vi "runTestScenario.vi"(8 "error in (no error)":errorcluster, 11 "ADC Channel0 Test  in":refnum<class "ADC Channel0 Test.lvclass">) -> (0 "error out":errorcluster, 1 "Result":T1, 2 "TestExecution":T2, 3 "ADC Channel0 Test  out":refnum<class "ADC Channel0 Test.lvclass">)   [LabVIEW 2015, in "ADC Channel0 Test.lvclass"]
uses:
  ADC Channel0 Test.lvclass
  Typedefs/TestExecution.ctl
  Typedefs/PassFailTest.ctl
  ADC Channel0 Test.lvclass/ADC Channel0 Test.ctl
  Typedefs/WriteDataFileInput.ctl
  Typedefs/TestScenarioTypes.ctl
  Typedefs/WriteLogMessageInput.ctl
  <userlib>/Common/ILC/ILC/ILC.lvclass/ILC.ctl
  Model/TestLog/ITestLog/ITestLog.lvclass
  Typedefs/ILCBTTypedefs.lvlib
  <userlib>/Common/ILC/ILC/ILC.lvclass
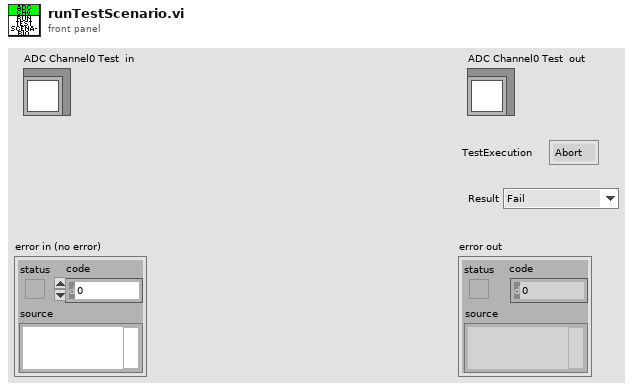
[diagram p1: front panel]
types:
  T1 = typedef "ILCBTTypedefs.lvlib/PassFailTest.ctl" = enum16{"Fail", "Pass", "NA"}
  T2 = typedef "ILCBTTypedefs.lvlib/TestExecution.ctl" = enum16{"Abort", "Continue"}
  T3 = typedef "ILCBTTypedefs.lvlib/WriteLogMessageInput.ctl" = cluster{"Test Scenario":T4, "Description":string, "Actual Value":string, "Data File":string, "Result":T1}
  T4 = typedef "ILCBTTypedefs.lvlib/TestScenarioTypes.ctl" = enum16{"+3.3VA Supply Test", "+3.3VD Supply Test", "+5VA Supply Test", "+5VD Supply Test", "Unique ID Test", "TEDS Status Test", "LIMSW1_TTL Low Test", "LIMSW1_TTL High Test", "LIMSW2_TTL Low Test", "LIMSW2_TTL High Test", "Tachometer Low Test", "Tachometer High Test", "SSR_TTL Low Test", "SSR_TTL High Test", "SM_GPI Low Test", "SM_GPI High Test", "CW Motion Without Limit Test", "CW Motion With Limit Test", "CW Motion With Both Limits Test", "CW Motion on CCW Limit Test", "CCW Motion Without Limit Test", "CCW Motion With Limit Test", "CCW Motion With Both Limits Test", "CCW Motion on CW Limit Test", "RS232-TXD Low Test", "RS232-TXD High Test", "RS232-RTS Low Test", "RS232-RTS High Test", "RS232-RXD Low Test", "RS232-RXD High Test", "RS232-CTS Low Test", "RS232-CTS High Test", "Out_SS Low Test", "Out_SS High Test", "Out_SDI Low Test", "Out_SDI High Test", "Out_SCLK Low Test", "Out_SCLK High Test", "Reset Low Test", "Reset High Test", "1 Channel ADC Test", "3 Channel ADC Test", "5 Channel ADC Test", "Vref Test", "ROT Test", "DAC1 Test", "DAC2 Test", "DAC3 Test", "DAC4 Test", "BIAS Test", "EXC1 Test", "EXC2 Test", "EXC3 Test", "EXC4 Test"}
  T5 = typedef "ILCBTTypedefs.lvlib/WriteDataFileInput.ctl" = cluster{"Test Scenario":T4, "File Name":string, "Output":string[]}
  T6 = typedef "ILCCommon.lvlib/ILCTypedefs.lvlib/InputData.ctl" = cluster{"Input Channels":T7, "Limit Switches":T8, "Tachometer":u16, "SSI Encoder":i32, "ADCs":T9}
  T7 = typedef "ILCCommon.lvlib/ILCConfiguration.lvlib/InputChannels.ctl" = enum16{"Channel 0", "3 Channels", "5 Channels"}
  T8 = typedef "ILCCommon.lvlib/ILCTypedefs.lvlib/LimitSwitches.ctl" = cluster{"1":bool, "2":bool}
  T9 = typedef "ILCCommon.lvlib/ILCTypedefs.lvlib/ADCs.ctl" = cluster{"Ch0":i32, "Ch1":i32, "Ch2":i32, "Ch3":i32, "Ch4":i32}
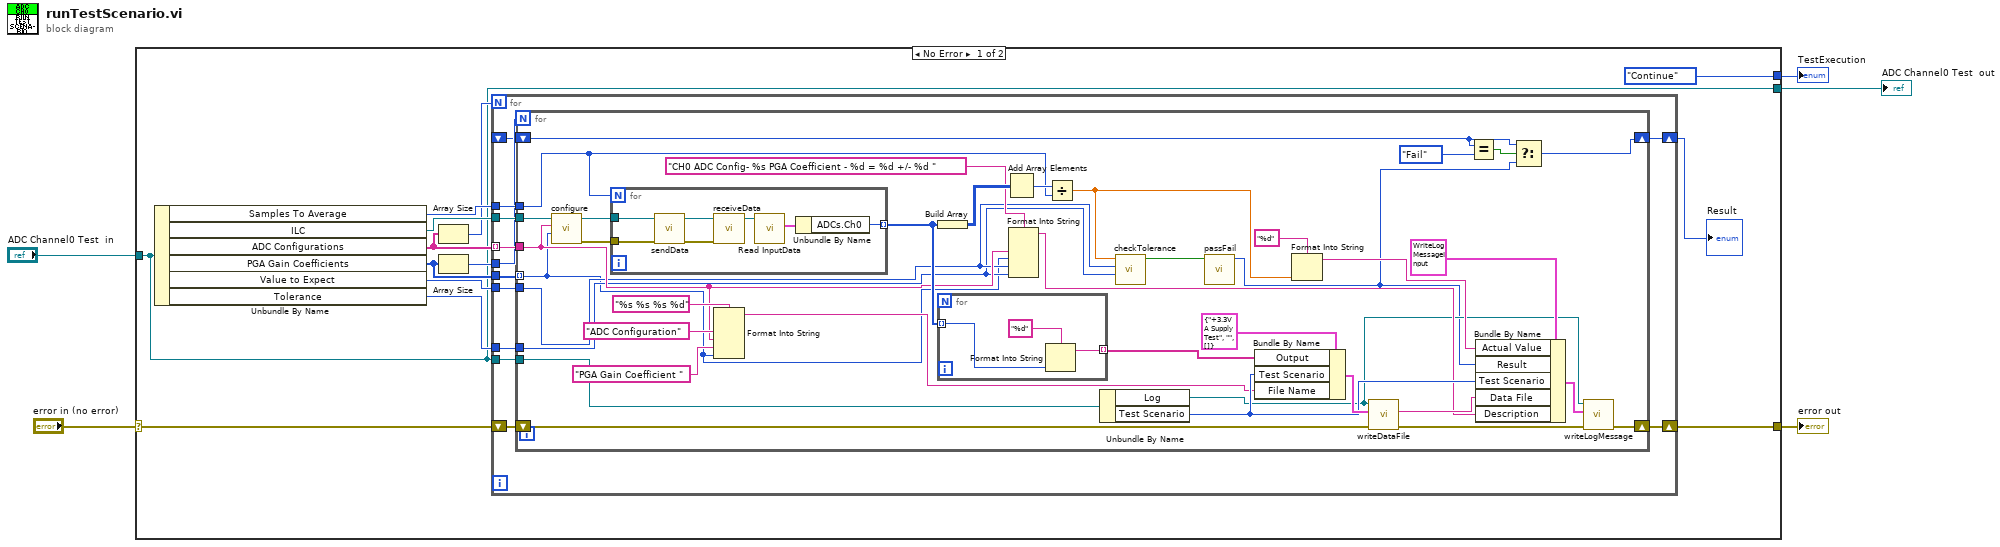
[diagram p0: block diagram]
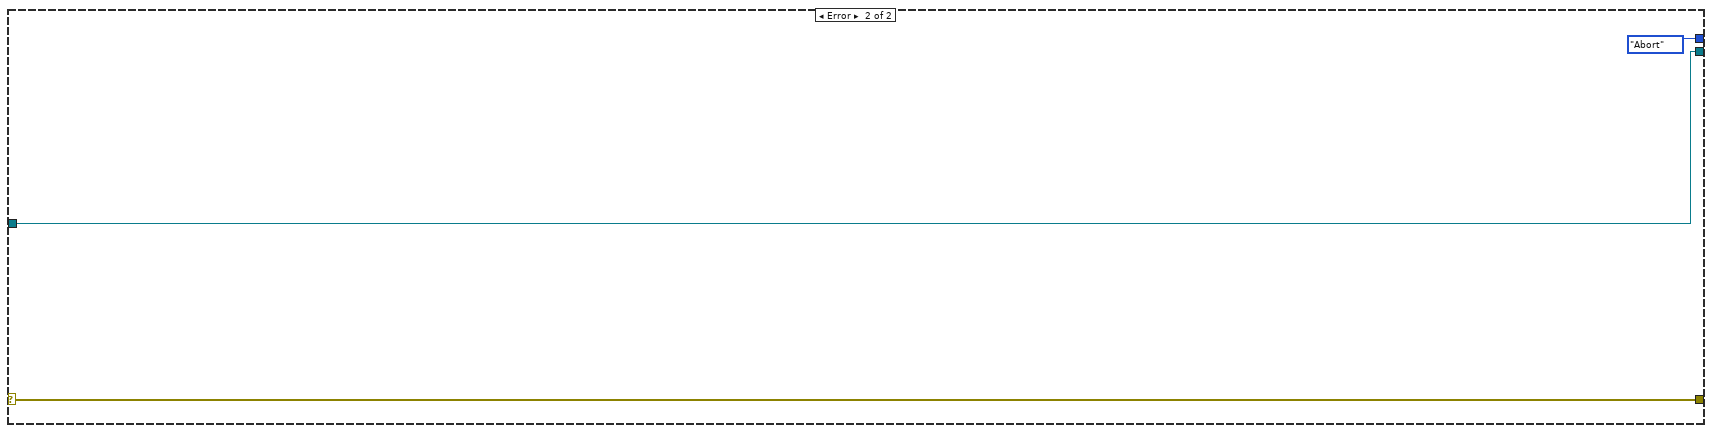
[diagram p2: hidden frame]
diagram:
  n1 = case shown="No Error" "error in (no error)" {
    selector: "error in (no error)" -> [w13 w81]
    tunnel: [w12 w81] -> w4
    tunnel: [TestExecution."Continue" ("TestExecution") TestExecution."Abort" ("TestExecution")] -> w3
    tunnel: "ADC Channel0 Test  in" -> [w7 w79]
    tunnel: [w7 w79] -> w1
    frame No Error {
      n2 = Unbundle By Name(w7) -> ("Samples To Average"=w16:i32, "ILC"=w18:refnum<class "ILC.lvclass">, "ADC Configurations"=w11:string[], "PGA Gain Coefficients"=w9:u16[], "Value to Expect"=w15:i32, "Tolerance"=w14:i32)
      n3 = Array Size(array=w11) -> (size(s)=w10:i32)
      n4 = Array Size(array=w9) -> (size(s)=w8:i32)
      n5 = for {
        N: w10 -> [_]
        tunnel: w18 -> [w30]
        tunnel: w9 -> [w21]
        tunnel: w16 -> [w29]
        tunnel: w7 -> [w28]
        tunnel: w15 -> [w27]
        tunnel: w14 -> [w26]
        tunnel: w11 -> [w23] mode=indexing
        shift-right: [w24] -> w12
        shift-left: w13 -> [w25]
        tunnel: w8 -> [w22]
        shift-right: [w20] -> w6
        shift-left: _ -> [w19]
        n6 = for {
          N: w22 -> [_]
          tunnel: w30 -> [w68]
          tunnel: w29 -> [w64]
          tunnel: w28 -> [w56]
          tunnel: w27 -> [w47]
          tunnel: w26 -> [w46]
          shift-right: [w37] -> w24
          shift-left: w25 -> [w39]
          tunnel: w23 -> [w48]
          tunnel: w21 -> [w36] mode=indexing
          shift-right: [w33] -> w20
          shift-left: w19 -> [w32]
          n7 = call <userlib>:"configure.vi"("PGA Gain"=w36, "ADC Configuration"=w48, "ILC in"=w68) -> ("error out"=w66:errorcluster, "ILC out"=w67:refnum<class "ILC.lvclass">)  [unwired: 7 in]
          n8 = for {
            N: w64 -> [_]
            tunnel: w67 -> [w78]
            tunnel: w66 -> [w77]
            tunnel: [w72] -> w55 mode=indexing
            n9 = call <userlib>:"sendData.vi"("error in (no error)"=w77, "ILC in"=w78) -> ("error out"=w76:errorcluster, "ILC out"=w75:refnum<class "ILC.lvclass">)  [unwired: 8 in]
            n10 = call <userlib>:"receiveData.vi"("error in (no error)"=w76, "ILC in"=w75) -> ("ILC out"=w73:refnum<class "ILC.lvclass">)  [unwired: 8 in, 1 out]
            n11 = call <userlib>:"Read InputData.vi"("ILC in"=w73) -> ("InputData"=w74:T6)  [unwired: 9 in, 1 out]
            n12 = Unbundle By Name(w74) -> ("ADCs.Ch0"=w72:i32)
          }
          n13 = Format Into String(format string="%s %s %s %d", "ADC Configuration" ("input 1"), w48, "PGA Gain Coefficient " ("initial string"), w36) -> (resulting string=w50:string)  [unwired: 2 in, 1 out]
          n14 = Build Array(w55) -> (w57:i32[][])
          n15 = for {
            tunnel: w55 -> [w71] mode=indexing
            tunnel: [w70] -> w54 mode=indexing
            n16 = Format Into String(format string="%d", w71) -> (resulting string=w70:string)  [unwired: 2 in, 1 out]
          }
          n17 = Add Array Elements(numeric array=w57) -> (sum=w65:i32)
          n18 = Format Into String(format string="CH0 ADC Config- %s PGA Coefficient - %d = %d +/- %d ", w48, w36, w47, w46) -> (resulting string=w45:string)  [unwired: 2 in, 1 out]
          n19 = Divide(x=w65, y=w64) -> (x/y=w44:dbl)
          n20 = Unbundle By Name(w56) -> ("Log"=w40:refnum<class "ITestLog.lvclass">, "Test Scenario"=w52:T4)
          n21 = call "checkTolerance.vi"("Tolerance"=w46, "Expected Value"=w47, "Average"=w44) -> ("Boolean"=w63:bool)  [unwired: 8 in]
          n22 = call "passFail.vi"("Boolean"=w63) -> ("Result"=w34:T1)  [unwired: 10 in]
          n23 = Bundle By Name(cluster=T5 {"Test Scenario"=enum."+3.3VA Supply Test", "File Name"="", "Output"=[]} ("WriteDataFileInput"), "Output"=w54, "Test Scenario"=w52, "File Name"=w50) -> (w58:T5)
          n24 = Format Into String(format string="%d", w44) -> (resulting string=w43:string)  [unwired: 2 in, 1 out]
          n25 = call-dynamic "writeDataFile.vi"("error in (no error)"=w39, "WriteDataFileInput"=w58, "ITestLog in"=w40) -> ("error out"=w38:errorcluster, "Relative Path"=w51:string)  [unwired: 6 in, 1 out]
          n26 = Equal?(x=w32, y=PassFailTest."Fail") -> (x = y?=w31:bool)
          n27 = Bundle By Name(cluster=T3 {"Test Scenario"=enum."+3.3VA Supply Test", "Description"="", "Actual Value"="", "Data File"="", "Result"=enum."Fail"} ("input cluster"), "Actual Value"=w43, "Result"=w34, "Test Scenario"=w52, "Data File"=w51, "Description"=w45) -> (w41:T3)
          n28 = Select(t=w32, s=w31, f=w34) -> (s? t:f=w33:T1)
          n29 = call-dynamic "writeLogMessage.vi"("error in (no error)"=w38, "WriteLogMessageInput"=w41, "ITestLog in"=w40) -> ("error out"=w37:errorcluster)  [unwired: 7 in, 1 out]
        }
      }
      "Result" <- w6
    }
    frame Error {
    }
  }
  "ADC Channel0 Test  out" <- w1
  "error out" <- w4
  "TestExecution" <- w3
